vi "Scan (To).vi"(8 "error in (no error)":errorcluster, 9 "Reference to a Stop button":refnum<vi>, 10 "END LAMBDA":dbl=100.0 min=0.0 max=16777215.000000011 step=0.010000000000000007 format="%.2f", 11 "VISA resource name":refnum<visa-resource-name>) -> (0 "error out":errorcluster, 3 "VISA resource name out":refnum<visa-resource-name>)   [LabVIEW 2009, in "Digikrom DK24x.lvlib"]
doc: "Scans the monochromator between the present position and a alternate specified wavelength, at a rate determined by the SPEED command. Valid values of position are grating dependent."
uses:
  Digikrom DK24x.lvlib
  Private/Command.ctl
panel:
  # "nm"
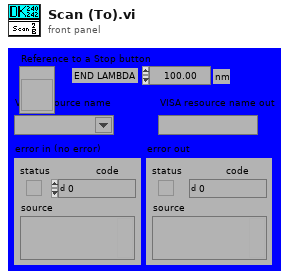
[diagram p1: front panel]
types:
  T1 = typedef "Digikrom DK24x.lvlib/Command.ctl" = u8
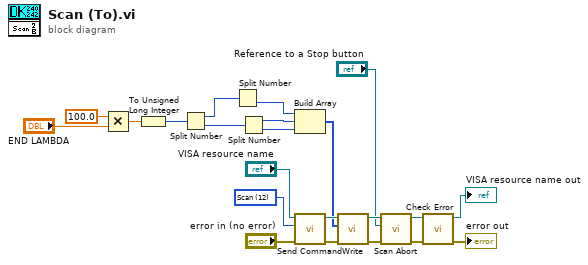
[diagram p0: block diagram]
diagram:
  w1 = T1 12 items=["Cancel"=24, "Clear"=25, "CSR"=28, "Echo"=27, "Filter"=15, "Gcal"=18, "Goto"=16, "Grtid?"=19, "Grtsel"=26, "NOVRAM Read"=56, "NOVRAM Write"=59, "Reset"=255, "Scan"=12, "Scan Up"=9, "Scan Down"=3, "Serial?"=33, "Slew Up"=8, "Slew Down"=2, "Slit Reset"=43, "Slit?"=30, "Sltadj"=14, "Speed"=13, "Sspeed?"=21, "Step Down"=1, "Step Up"=7, "S1adj"=31, "S2adj"=32, "S3adj"=34, "S1cal"=22, "S2cal"=23, "S3cal"=35, "Test"=17, "Type"=57, "Wave?"=29, "Zero"=52] ("Command")
  n1 = Multiply(x=100.0, y="END LAMBDA") -> (x*y=w18:dbl)
  n2 = To Unsigned Long Integer(number=w18) -> (unsigned 32bit integer=w17:u32)
  n3 = Split Number(x=w17) -> (hi(x)=w16:u16, lo(x)=w15:u16)
  n4 = Split Number(x=w16) -> (lo(x)=w14:u8)  [unwired: 1 out]
  n5 = Split Number(x=w15) -> (hi(x)=w13:u8, lo(x)=w12:u8)
  n6 = Build Array(w14, w13, w12) -> (w6:u8[])
  n7 = call "Send Command.vi"("error in (no error)"="error in (no error)", "Command"=w1, "VISA resource name"="VISA resource name") -> ("error out"=w7:errorcluster, "VISA resource name out"=w11:refnum<visa-resource-name>)  [unwired: 7 out]
  n8 = call "Write.vi"("error in (no error)"=w7, "Byte Array"=w6, "VISA resource name"=w11) -> ("error out"=w3:errorcluster, "VISA resource name out"=w10:refnum<visa-resource-name>)  [unwired: 7 out]
  n9 = call "Scan Abort.vi"("error in (no error)"=w3, "Reference to a Stop button"="Reference to a Stop button", "VISA resource name"=w10) -> ("error out"=w2:errorcluster, "VISA resource name out"=w5:refnum<visa-resource-name>)  [unwired: 7 out]
  n10 = call "Check Error.vi"("error in"=w2, "VISA resource name in"=w5) -> ("error out"=→"error out":errorcluster, "VISA resource name out"=→"VISA resource name out":refnum<visa-resource-name>)  [unwired: 1 in, 7 out]
